vi "Fresh Image.vi"(8 "error in (no error)":errorcluster, 11 "Actor in":refnum<class "Actor.lvclass">) -> (0 "error out":errorcluster, 3 "Actor out":refnum<class "Actor.lvclass">)   [LabVIEW 2015, in "Actor.lvclass"]
uses:
  Actor.lvclass
  Actor.lvclass/Actor.ctl
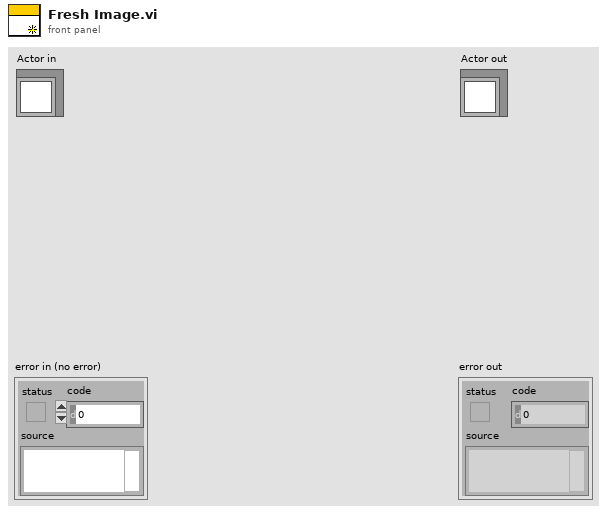
[diagram p1: front panel]
types:
  T1 = enum8{"Enabled", "Disabled", "Disabled and Grayed Out"}
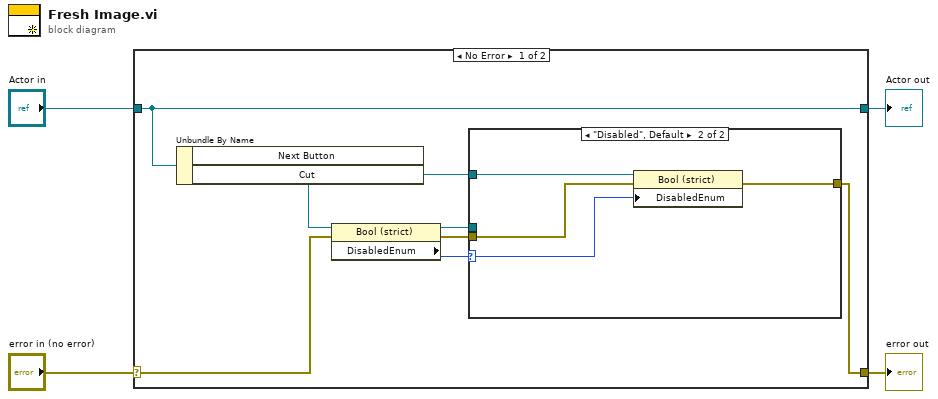
[diagram p0: block diagram]
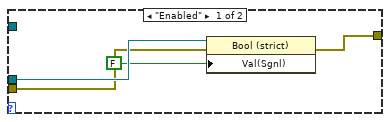
[diagram p2: hidden frame]
diagram:
  n1 = case shown="No Error" "error in (no error)" {
    selector: "error in (no error)" -> [w7 w22]
    tunnel: [w6 w22] -> w3
    tunnel: [w12 w21] -> w1
    tunnel: "Actor in" -> [w12 w21]
    frame No Error {
      n2 = Unbundle By Name(w12) -> ("Next Button"=w11:refnum<vi>, "Cut"=w5:refnum<vi>)
      n3 = property class="Bool (strict)"(reference=w11, error in=w7) -> (reference out=w9:refnum<vi>, error out=w8:errorcluster, "DisabledEnum"=w10:T1)
      n4 = case shown="\"Disabled\", Default" w10 {
        selector: w10 -> [_ w18]
        tunnel: w9 -> [w16 _]
        tunnel: w8 -> [w15 w19]
        tunnel: [w13 w17] -> w6
        tunnel: w5 -> [_ w20]
        frame "Enabled" {
          n5 = property class="Bool (strict)"(reference=w16, error in=w15, "Val(Sgnl)"=FALSE ("Value (Signaling)")) -> (error out=w13:errorcluster)  [unwired: 1 out]
        }
        frame "Disabled", Default {
          n6 = property class="Bool (strict)"(reference=w20, error in=w19, "DisabledEnum"=w18) -> (error out=w17:errorcluster)  [unwired: 1 out]
        }
      }
    }
    frame Error {
    }
  }
  "error out" <- w3
  "Actor out" <- w1
